vi "strain_Q.vi"(7 "cmd":enum16{"create", "write", "read", "close"}(ring), 8 "error in":errorcluster, 11 "data":enum16{"run", "stop", "close"}(ring)) -> (0 "error out":errorcluster, 3 "queue out":refnum<queue>)   [LabVIEW 2013]
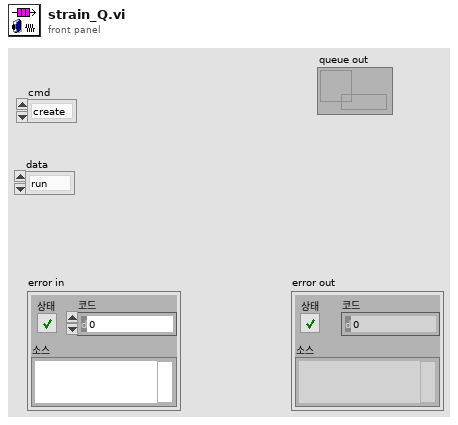
[diagram p1: front panel]
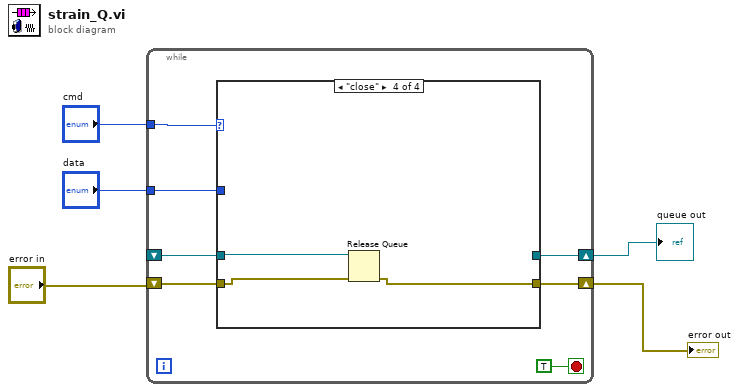
[diagram p0: block diagram]
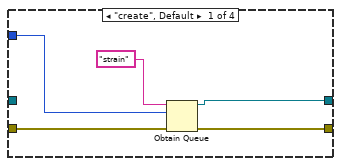
[diagram p2: hidden frame]
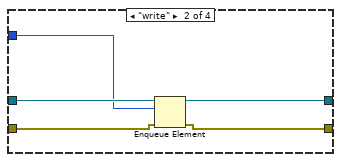
[diagram p3: hidden frame]
diagram:
  n1 = while {
    shift-right: [w12] -> w4
    shift-left: "error in" -> [w11]
    tunnel: "cmd" -> [w10]
    shift-right: [w9] -> w1
    shift-left: _ -> [w8]
    tunnel: "data" -> [w7]
    stop <- TRUE stop-if-true
    n2 = case shown="\"close\"" w10 {
      tunnel: [w16 w21 w24 w26] -> w12
      tunnel: w11 -> [w17 w22 w24 w27]
      tunnel: [w14 w20 w23 _] -> w9
      tunnel: w8 -> [_ w19 w23 w25]
      tunnel: w7 -> [w13 w18 _ _]
      frame "create", Default {
        n3 = Obtain Queue(name (unnamed)="strain" ("이름(이름없음)"), element data type=w13, error in (no error)=w17) -> (queue out=w14:refnum<queue>, error out=w16:errorcluster)  [unwired: 2 in, 1 out]
      }
      frame "write" {
        n4 = Enqueue Element(queue=w19, element=w18, error in (no error)=w22) -> (queue out=w20:refnum<queue>, error out=w21:errorcluster)  [unwired: 1 in, 1 out]
      }
      frame "read" {
      }
      frame "close" {
        n5 = Release Queue(queue=w25, error in (no error)=w27) -> (error out=w26:errorcluster)  [unwired: 1 in, 2 out]
      }
    }
  }
  "error out" <- w4
  "queue out" <- w1
